vi "New Double Group.vi"(8 "error in (no error)":errorcluster, 10 "Group Config":refnum<class "Group Config.lvclass">, 11 "ChannelService in":refnum<class "ChannelService.lvclass">) -> (0 "error out":errorcluster, 2 "Group":refnum<class "Group.lvclass">, 3 "ChannelService out":refnum<class "ChannelService.lvclass">)   [LabVIEW 2020, in "Vecto.lvlib" / "ChannelService.lvclass"]
uses:
  ChannelService.lvclass
  Group/Group.lvclass
  C:/dev/lv20CE/relink/lv-vecto/Vecto/GroupAbstract/GroupAbstract.lvclass
  Group Config/Group Config.lvclass
  ChannelService.lvclass/ChannelService.ctl
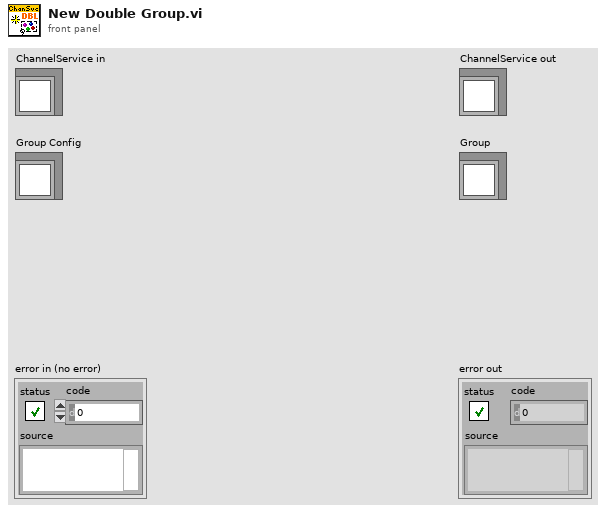
[diagram p1: front panel]
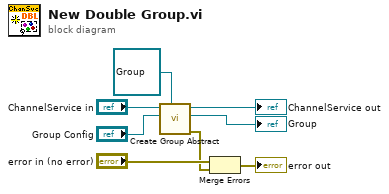
[diagram p0: block diagram]
diagram:
  n1 = call "Create Group Abstract.vi"("Group Type"=refnum<class "Group.lvclass"> refnum ("Group"), "Group Config"="Group Config", "ChannelService in"="ChannelService in") -> ("error out"=w2:errorcluster, "Group"=→"Group":refnum<class "Group.lvclass">, "ChannelService out"=→"ChannelService out":refnum<class "ChannelService.lvclass">)  [unwired: 6 in]
  n2 = Merge Errors("error in (no error)", w2) -> (→"error out":errorcluster)
